vi "LH_ECD.vi"(0 "FPGA-VI-Referenz (Ausgang)":refnum<k20>, 1 "OutputRange":cluster{"output high":dbl, "output low":dbl}[](array[cluster]), 2 "LHSetpoints":dbl[](array[numeric]), 3 "AIsLH":i32[](array[numeric]), 4 "error in":errorcluster, 5 "LH-Gruppe":bool[](array[boolean])=[FALSE, FALSE, FALSE, FALSE, FALSE, FALSE, FALSE, FALSE, FALSE, FALSE, FALSE, FALSE], 6 "PIDs für \"träge\" Heizungen":T1(array[cluster])) -> (7 "error out":errorcluster)   [LabVIEW 2017]
uses:
  GVAIs_ECD.vi
  <vilib>/addons/control/pid/pid.llb/PID (DBL Array).vi
  <vilib>/Utility/error.llb/Error Cluster From Error Code.vi
  <vilib>/rvi/errors/niLvFpgaAdjustHostInterfaceError.vi
  <vilib>/rvi/interface/nirviReadWriteControl/nirviReadWriteControl.xnode
  FPGA Bitfiles/HAGAR-V_FPGATargetECD_FPGA-ProgrammECD_LbBtUh8SPQY.lvbitx
  FPGA_ECD/FPGA-Programm_ECD.vi
  <vilib>/addons/control/pid/NI_PID_pid.lvlib
  NiFpgaLv.dll
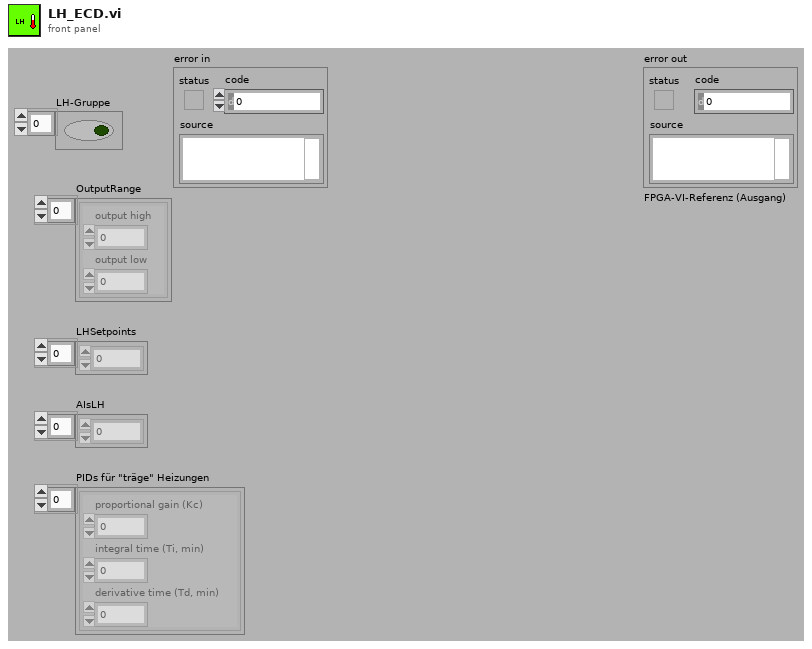
[diagram p1: front panel]
types:
  T1 = cluster{"proportional gain (Kc)":dbl, "integral time (Ti, min)":dbl, "derivative time (Td, min)":dbl}[]
  T2 = cluster{"[0]":bool, "[1]":bool, "[2]":bool, "[3]":bool, "[4]":bool, "[5]":bool, "[6]":bool, "[7]":bool, "[8]":bool, "[9]":bool, "[10]":bool, "[11]":bool, "[12]":bool}
  T3 = cluster{"[0]":u32, "[1]":u32, "[2]":u32, "[3]":u32, "[4]":u32, "[5]":u32, "[6]":u32, "[7]":u32, "[8]":u32, "[9]":u32, "[10]":u32, "[11]":u32, "[12]":u32}
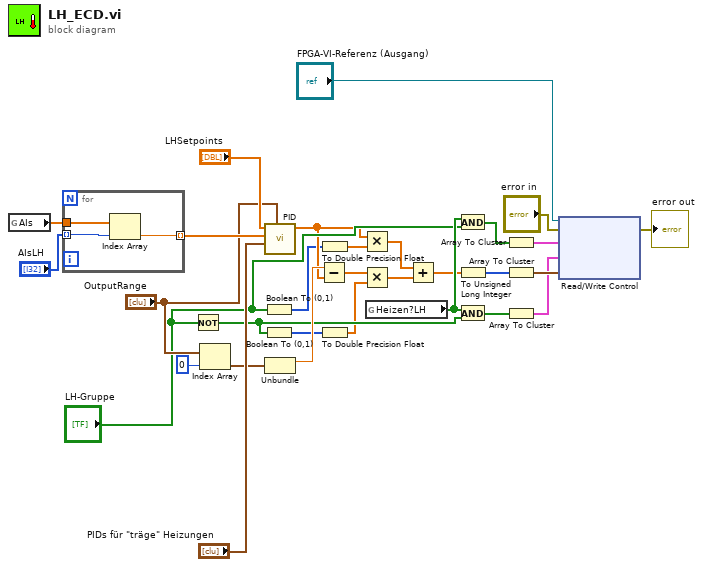
[diagram p0: block diagram]
diagram:
  n1 = global read "GVAIs_ECD.vi" "AIs"() -> (w28:dbl[])
  n2 = for {
    tunnel: w28 -> [w33]
    tunnel: "AIsLH" -> [w32] mode=indexing
    tunnel: [w31] -> w24 mode=indexing
    n3 = Index Array(array=w33, index=w32) -> (element=w31:dbl)
  }
  n4 = Not(x="LH-Gruppe") -> (.not. x?=w3:bool[])
  n5 = Index Array(array="OutputRange", index=0) -> (element=w15:cluster{"output high":dbl, "output low":dbl})
  n6 = Boolean To (0,1)(Boolean="LH-Gruppe") -> (0, 1=w11:i16[])
  n7 = Boolean To (0,1)(Boolean=w3) -> (0, 1=w4:i16[])
  n8 = call-poly <vilib>:"PID.vi"("output range"="OutputRange", "PID gains"="PIDs für \"träge\" Heizungen", "process variable"=w24, "setpoint"="LHSetpoints") -> ("output"=w12:dbl[])  [unwired: 6 in, 1 out]
  n9 = Unbundle(w15) -> ("output high"=w13:dbl)  [unwired: 1 out]
  n10 = Subtract(x=w13, y=w12) -> (x-y=w10:dbl[])
  n11 = To Double Precision Float(number=w11) -> (double precision float=w5:dbl[])
  n12 = To Double Precision Float(number=w4) -> (double precision float=w2:dbl[])
  n13 = Multiply(x=w12, y=w5) -> (x*y=w9:dbl[])
  n14 = Multiply(x=w10, y=w2) -> (x*y=w8:dbl[])
  n15 = global read "GVHeizenLH_ECD.vi" "Heizen?LH"() -> (w20:bool[])
  n16 = Add(x=w9, y=w8) -> (x+y=w7:dbl[])
  n17 = And(x=w20, y="LH-Gruppe") -> (x .and. y?=w21:bool[])
  n18 = To Unsigned Long Integer(number=w7) -> (unsigned 32bit integer=w6:u32[])
  n19 = And(x=w20, y=w3) -> (x .and. y?=w19:bool[])
  n20 = Array To Cluster(array=w21) -> (cluster=w22:T2)
  n21 = Array To Cluster(array=w6) -> (cluster=w23:T3)
  n22 = Array To Cluster(array=w19) -> (cluster=w18:T2)
  n23 = xnode "Read/Write Control"("FPGA-VI-Referenz (Eingang)"="FPGA-VI-Referenz (Ausgang)", "Fehler (Eingang)"="error in", "LHHeizen1?"=w22, "LHHeizen2?"=w18, "LHPulse(us)"=w23) -> ("Fehler (Ausgang)"=→"error out":errorcluster)  [unwired: 1 out]
